vi "SL Write Multiple Tags.vi"(8 "error in (no error)":errorcluster, 9 "timestamp":timestamp, 10 "Values":dbl[](array[numeric]), 11 "SkyLine.Refs":refnum<class "NI Skyline Tag.lvclass">[](array[class])) -> (0 "error out":errorcluster)   [LabVIEW 2019, in "Data Publishing Service.lvlib"]
uses:
  Data Publishing Service.lvlib
  <vilib>/Skyline/Tag/Wrapper/Wrapper_class/NI Skyline Tag.lvclass
  <vilib>/Skyline/Tag/Shared/typedefs/DataType.ctl
  <vilib>/Skyline/Tag/Shared/NI Skyline Tag.lvlib
  <vilib>/Skyline/Tag/Shared/typedefs/Tag Value Cluster.ctl
  <vilib>/Skyline/Configuration/Configuration_class/NI Skyline Configuration.lvclass
  <vilib>/Skyline/Tag/Wrapper/Wrapper_class/Tag Value Cluster Wrapper.ctl
  <vilib>/Skyline/Tag/Wrapper/Wrapper_class/Generate Tag Cluster (DBL) 2.vi
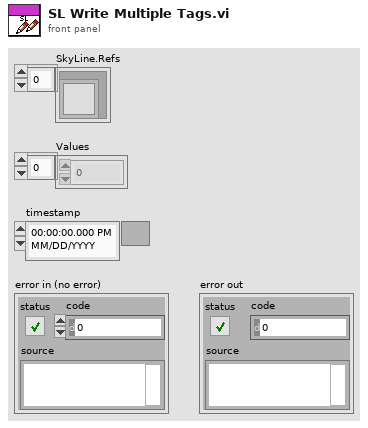
[diagram p1: front panel]
types:
  T1 = typedef "NI Skyline Tag.lvclass/Tag Value Cluster Wrapper.ctl" = cluster{"Configuration":refnum<class "NI Skyline Configuration.lvclass">, "Tag Cluster":T2}
  T2 = typedef "NI Skyline Tag.lvlib/Tag Value Cluster.ctl" = cluster{"Path":string, "Data Type":T3, "Value":string, "Time Stamp":timestamp}
  T3 = typedef "NI Skyline Tag.lvlib/DataType.ctl" = enum32{"Double", "I32", "String", "Boolean", "U64", "Timestamp"}
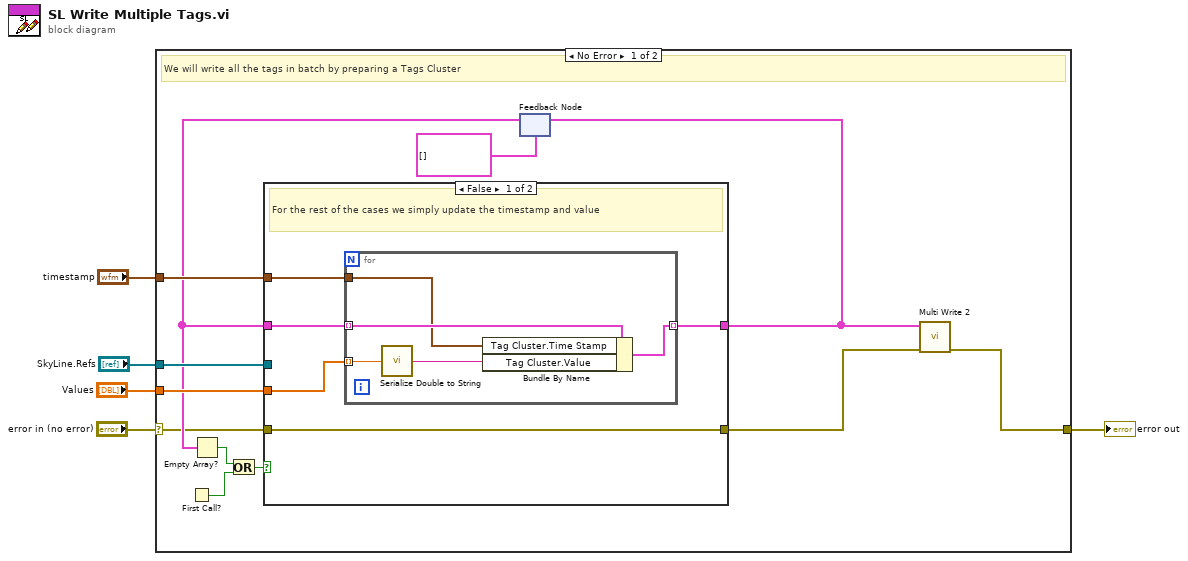
[diagram p0: block diagram]
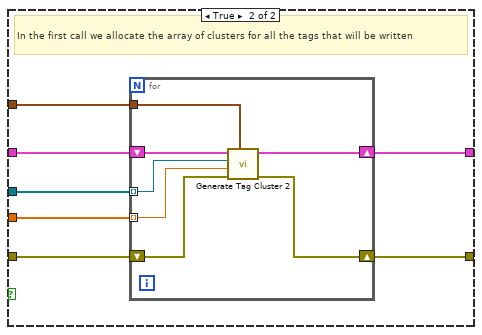
[diagram p2: hidden frame]
diagram:
  n1 = case shown="No Error" "error in (no error)" {
    selector: "error in (no error)" -> [w7 w42]
    tunnel: "SkyLine.Refs" -> [w17 _]
    tunnel: "Values" -> [w16 _]
    tunnel: "timestamp" -> [w15 _]
    tunnel: [w6 w42] -> w1
    frame No Error {
      # "We will write all the tags in batch by preparing a Tags Cluster"
      n2 = First Call?() -> (First Call?: T/F=w10:bool)
      n3 = feedback #1(T1[] [] ("tag clusters in")) -> (w13:T1[])
      n4 = Empty Array?(array=w13) -> (empty?=w11:bool)
      n5 = Or(x=w11, y=w10) -> (x .or. y?=w12:bool)
      n6 = case shown="False" w12 {
        tunnel: w17 -> [_ w34]
        tunnel: w16 -> [w18 w33]
        tunnel: w7 -> [w22 w32]
        tunnel: w15 -> [w19 w31]
        tunnel: [w22 w30] -> w8
        tunnel: [w20 w29] -> w9
        tunnel: w13 -> [w21 w28]
        frame False {
          # "For the rest of the cases we simply update the timestamp and value"
          n7 = for {
            tunnel: w21 -> [w27] mode=indexing
            tunnel: [w26] -> w20 mode=indexing
            tunnel: w19 -> [w25]
            tunnel: w18 -> [w23] mode=indexing
            n8 = call <vilib>:"Serialize Double to String.vi"("double"=w23) -> ("string"=w24:string)
            n9 = Bundle By Name(cluster=w27, "Tag Cluster.Time Stamp"=w25, "Tag Cluster.Value"=w24) -> (w26:T1)
          }
        }
        frame True {
          # "In the first call we allocate the array of clusters for all the tags that will be written"
          n10 = for {
            shift-right: [w37] -> w29
            shift-left: w28 -> [w41]
            tunnel: w34 -> [w40] mode=indexing
            tunnel: w33 -> [w39] mode=indexing
            shift-right: [w35] -> w30
            shift-left: w32 -> [w38]
            tunnel: w31 -> [w36]
            n11 = call-poly <vilib>:"Generate Tag Cluster 2.vi"("time stamp"=w36, "error in (no error)"=w38, "value"=w39, "tag in"=w40, "tag clusters in"=w41) -> ("error out"=w35:errorcluster, "tag clusters out"=w37:T1[])  [unwired: 4 in, 1 out]
          }
        }
      }
      n12 = feedback-in #1(w9) -> ()
      n13 = call <vilib>:"Multi Write 2.vi"("error in (no error)"=w8, "tag clusters"=w9) -> ("error out"=w6:errorcluster)  [unwired: 9 in]
    }
    frame Error {
    }
  }
  "error out" <- w1
